vi "SequenceFile Simple Execute.vi"() -> ()   [LabVIEW 2020]
uses:
  Engine/Engine.lvclass
  SequenceFile/SequenceFile.lvclass
panel:
  in  "Entry Point":string(combo)="Single Pass"
  out "Status":string
  in  "SequenceFile Path":path=path "C:/Users/Public/Documents/National Instruments/TestStand 2019 (32-bit)/Examples/Demos/Computer Motherboard Test/LabVIEW/Computer Motherboard Test Sequence.seq"
  # "1."
  # "2."
  # "1. Select the sequence file you'd like to run.\n\n2. Enter the name of the entry point to use in the process model. This is usually 'Test UUTs' or 'Single Pass' for models that ship with TestStand."
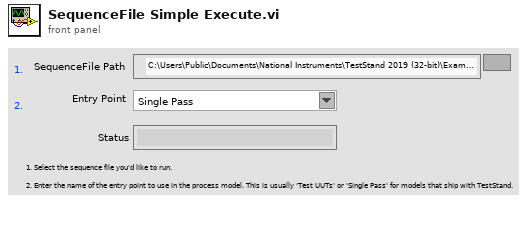
[diagram p1: front panel]
types:
  T1 = typedef "TSS.lvlib/Engine.lvclass/Session Handle.ctl" = refnum<data-value>
  T2 = typedef "TSS.lvlib/SequenceFile.lvclass/Session Handle.ctl" = refnum<data-value>
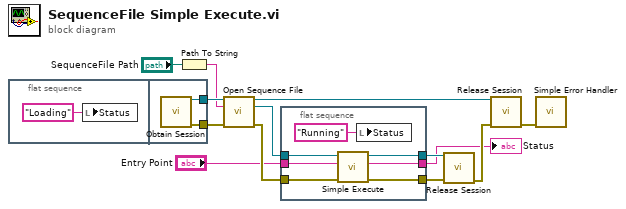
[diagram p0: block diagram]
diagram:
  n1 = flat-sequence {
    tunnel: [w16] -> w12
    tunnel: [w15] -> w10
    frame #0 {
      n2 = local write "Status"("Loading" ("Status")) -> ()
    }
    frame #1 {
      n3 = call "Obtain Session.vi"() -> ("Session Handle"=w16:T1, "error out"=w15:errorcluster)  [unwired: 14 in]
    }
  }
  n4 = Path To String(path="SequenceFile Path") -> (string=w9:string)
  n5 = call "Open Sequence File.vi"("Session Handle in"=w12, "File Path"=w9, "error in (no error)"=w10) -> ("Session Handle out"=w1:T1, "SequenceFile"=w7:T2, "error out"=w6:errorcluster)  [unwired: 10 in]
  n6 = flat-sequence {
    tunnel: w7 -> [w23]
    tunnel: w6 -> [w22]
    tunnel: "Entry Point" -> [w21]
    tunnel: [w20] -> w4
    tunnel: [w19] -> w3
    tunnel: [w18] -> w2
    frame #0 {
      n7 = call "Simple Execute.vi"("error in (no error)"=w22, "Entry Point / Sequence"=w21, "Session Handle in"=w23) -> ("error out"=w19:errorcluster, "Status"=w18:string, "Session Handle out"=w20:T2)  [unwired: 5 in, 1 out]
      n8 = local write "Status"("Running" ("Status")) -> ()
    }
  }
  n9 = call "Release Session.vi"("Session Handle"=w4, "error in (no error)"=w3) -> ("error out"=w13:errorcluster)  [unwired: 13 in]
  n10 = call "Release Session.vi"("Session Handle"=w1, "error in (no error)"=w13) -> ("error out"=w8:errorcluster)  [unwired: 13 in]
  n11 = call <vilib>:"Simple Error Handler.vi"("error in (no error)"=w8) -> ()  [unwired: 4 in, 5 out]
  "Status" <- w2
